vi "Framework.Create.Plugins.vi"(8 "error in (no error)":errorcluster, 10 "Plugin Configurations":refnum<class "Plugin Configuration.lvclass">[](array[class]), 11 "Framework in":refnum<class "Framework.lvclass">) -> (0 "error out":errorcluster, 2 "Plugins":refnum<class "Plugin.lvclass">[](array[class]), 3 "Framework out":refnum<class "Framework.lvclass">)   [LabVIEW 2017, in "DSF Core.lvlib" / "Framework.lvclass"]
uses:
  Framework.lvclass
  Shared/Classes/Plugin/Plugin Configuration.lvclass
  Plugin/Plugin.lvclass
  Framework.lvclass/Framework.ctl
  Shared/Classes/Plugin/Plugin Configuration.lvclass/Plugin Configuration.ctl
  Component Loader/Component Loader.lvclass
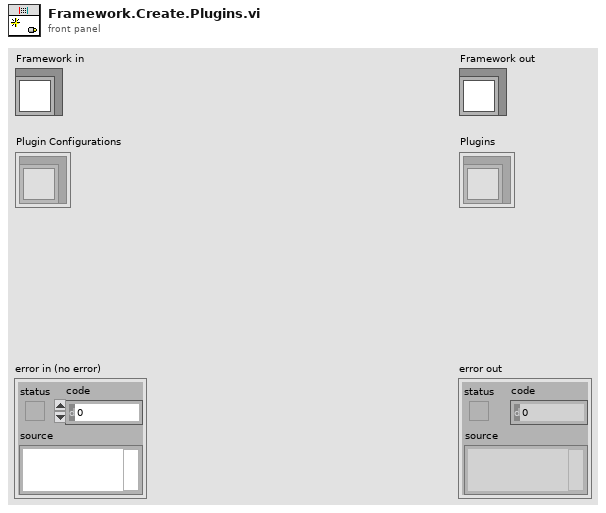
[diagram p1: front panel]
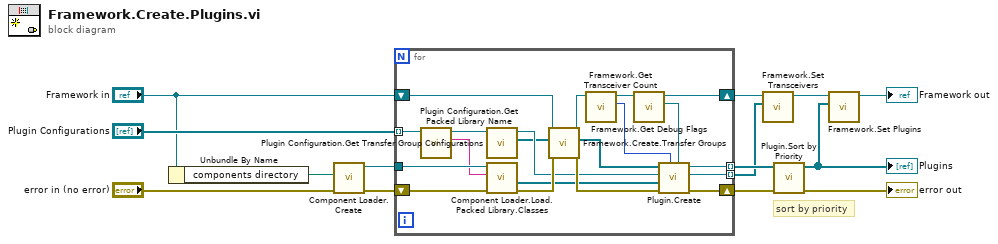
[diagram p0: block diagram]
diagram:
  # "sort by priority"
  n1 = Unbundle By Name("Framework in") -> ("components directory"=w3:path)
  n2 = call "Component Loader.Create.vi"("error in (no error)"="error in (no error)", "components directory"=w3) -> ("error out"=w4:errorcluster, "Component Loader out"=w6:refnum<class "Component Loader.lvclass">)  [unwired: 8 in]
  n3 = for {
    shift-right: [w32] -> w13
    shift-left: w4 -> [w17]
    shift-right: [w28] -> w9
    shift-left: "Framework in" -> [w31]
    tunnel: "Plugin Configurations" -> [w26] mode=indexing
    tunnel: [w30] -> w11 mode=indexing
    tunnel: w6 -> [w24]
    tunnel: [w21] -> w5 mode=indexing
    n4 = call "Plugin Configuration.Get Packed Library Name.vi"("Plugin Configuration in"=w26) -> ("packed library name"=w23:string, "Plugin Configuration out"=w25:refnum<class "Plugin Configuration.lvclass">)  [unwired: 9 in]
    n5 = call "Plugin Configuration.Get Transfer Group Configurations.vi"("Plugin Configuration in"=w25) -> ("Transfer Group Configurations"=w15:refnum<class "Transfer Group Configuration.lvclass">[], "Plugin Configuration out"=w16:refnum<class "Plugin Configuration.lvclass">)  [unwired: 9 in]
    n6 = call "Component Loader.Load.Packed Library.Classes.vi"("error in (no error)"=w17, "packed library name"=w23, "Component Loader in"=w24) -> ("error out"=w33:errorcluster, "objects"=w19:refnum<class>[])  [unwired: 6 in, 1 out]
    n7 = call "Framework.Create.Transfer Groups.vi"("error in (no error)"=w33, "Transfer Group Configurations"=w15, "Framework in"=w31) -> ("error out"=w34:errorcluster, "Transfer Groups"=w18:refnum<class "Transfer Group.lvclass">[], "Framework out"=w29:refnum<class "Framework.lvclass">)  [unwired: 6 in]
    n8 = call "Framework.Get Transceiver Count.vi"("Framework in"=w29) -> ("transceiver count"=w22:i32, "Framework out"=w27:refnum<class "Framework.lvclass">)  [unwired: 9 in]
    n9 = call "Framework.Get Debug Flags.vi"("Framework in"=w27) -> ("Debug Flags"=w20:refnum<class "Debug Flags.lvclass">, "Framework out"=w28:refnum<class "Framework.lvclass">)  [unwired: 9 in]
    n10 = call "Plugin.Create.vi"("Debug Flags"=w20, "transceiver count"=w22, "error in (no error)"=w34, "component classes"=w19, "Plugin Configuration"=w16, "Transfer Groups"=w18) -> ("error out"=w32:errorcluster, "Transceiver"=w21:refnum<class "Transceiver.lvclass">, "Plugin out"=w30:refnum<class "Plugin.lvclass">)  [unwired: 3 in]
  }
  n11 = call "Framework.Set Transceivers.vi"("Transceivers"=w5, "Framework in"=w9) -> ("Framework out"=w8:refnum<class "Framework.lvclass">)  [unwired: 9 in]
  n12 = call "Plugin.Sort by Priority.vi"("error in (no error)"=w13, "Plugins in"=w11) -> ("error out"=→"error out":errorcluster, "Plugins out"=w10:refnum<class "Plugin.lvclass">[])  [unwired: 8 in]
  "Plugins" <- w10
  n13 = call "Framework.Set Plugins.vi"("Plugins"=w10, "Framework in"=w8) -> ("Framework out"=→"Framework out":refnum<class "Framework.lvclass">)  [unwired: 9 in]
